vi "Label Generation.vi"(8 "error in":errorcluster, 10 "Resistance Value":string[](array[string]), 11 "Serial No":string) -> (0 "error out":errorcluster, 1 "Print Data":T1, 2 "Printer Command":string, 3 "QR data":string, 4 "error out 2":errorcluster)   [LabVIEW 2021]
uses:
  Gen fgv action.ctl
panel:
  out "Printer Command Out":string
  out "bytes written":i32
  in  "error in (no error)":errorcluster
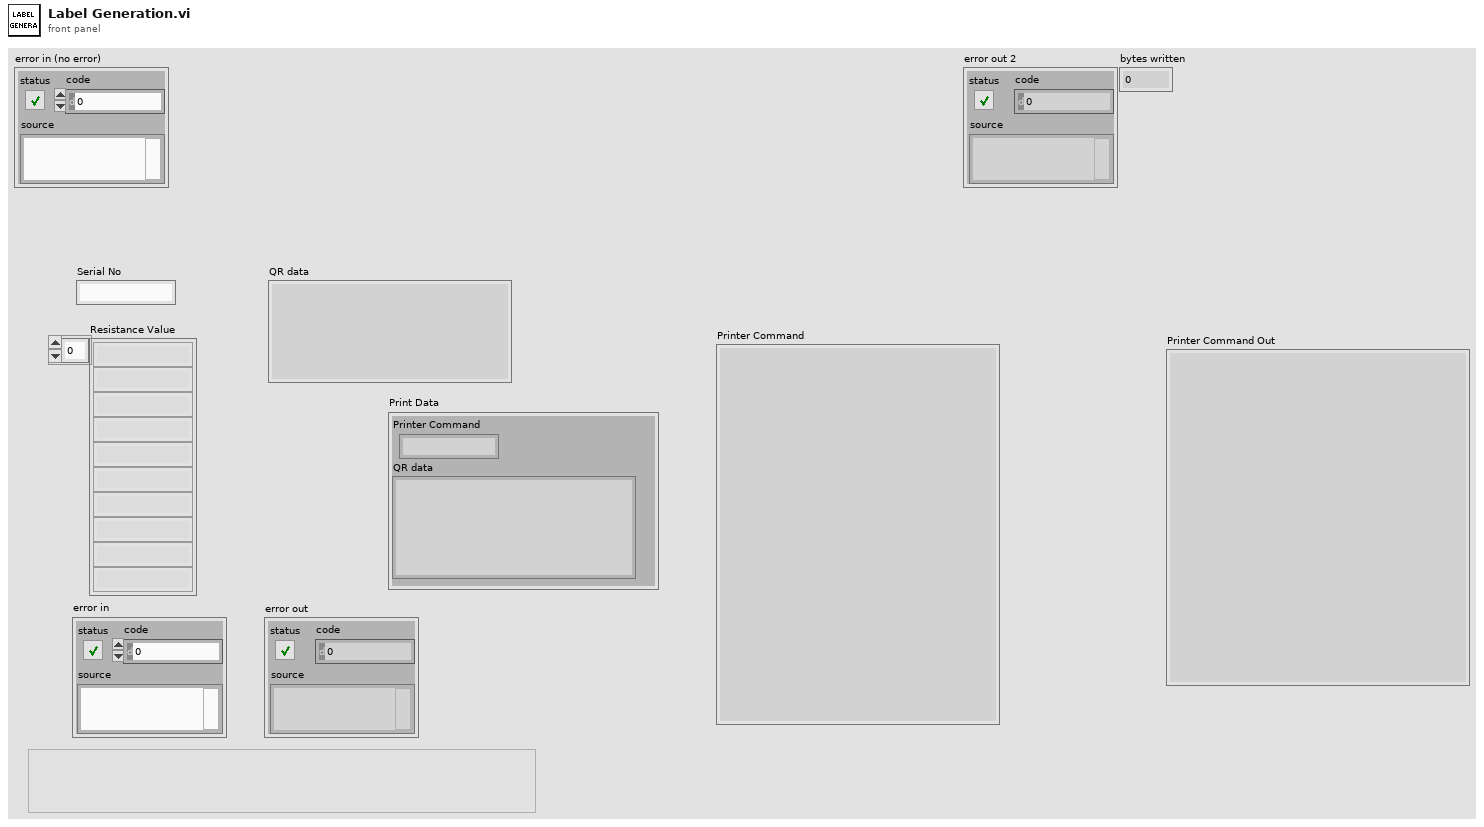
[diagram p1: front panel]
types:
  T1 = cluster{"Printer Command":string, "QR data":string}
  T2 = typedef "Gen FGV Action.ctl" = enum16{"Initialize", "Get Data", "Update Data", "Clear Data"}
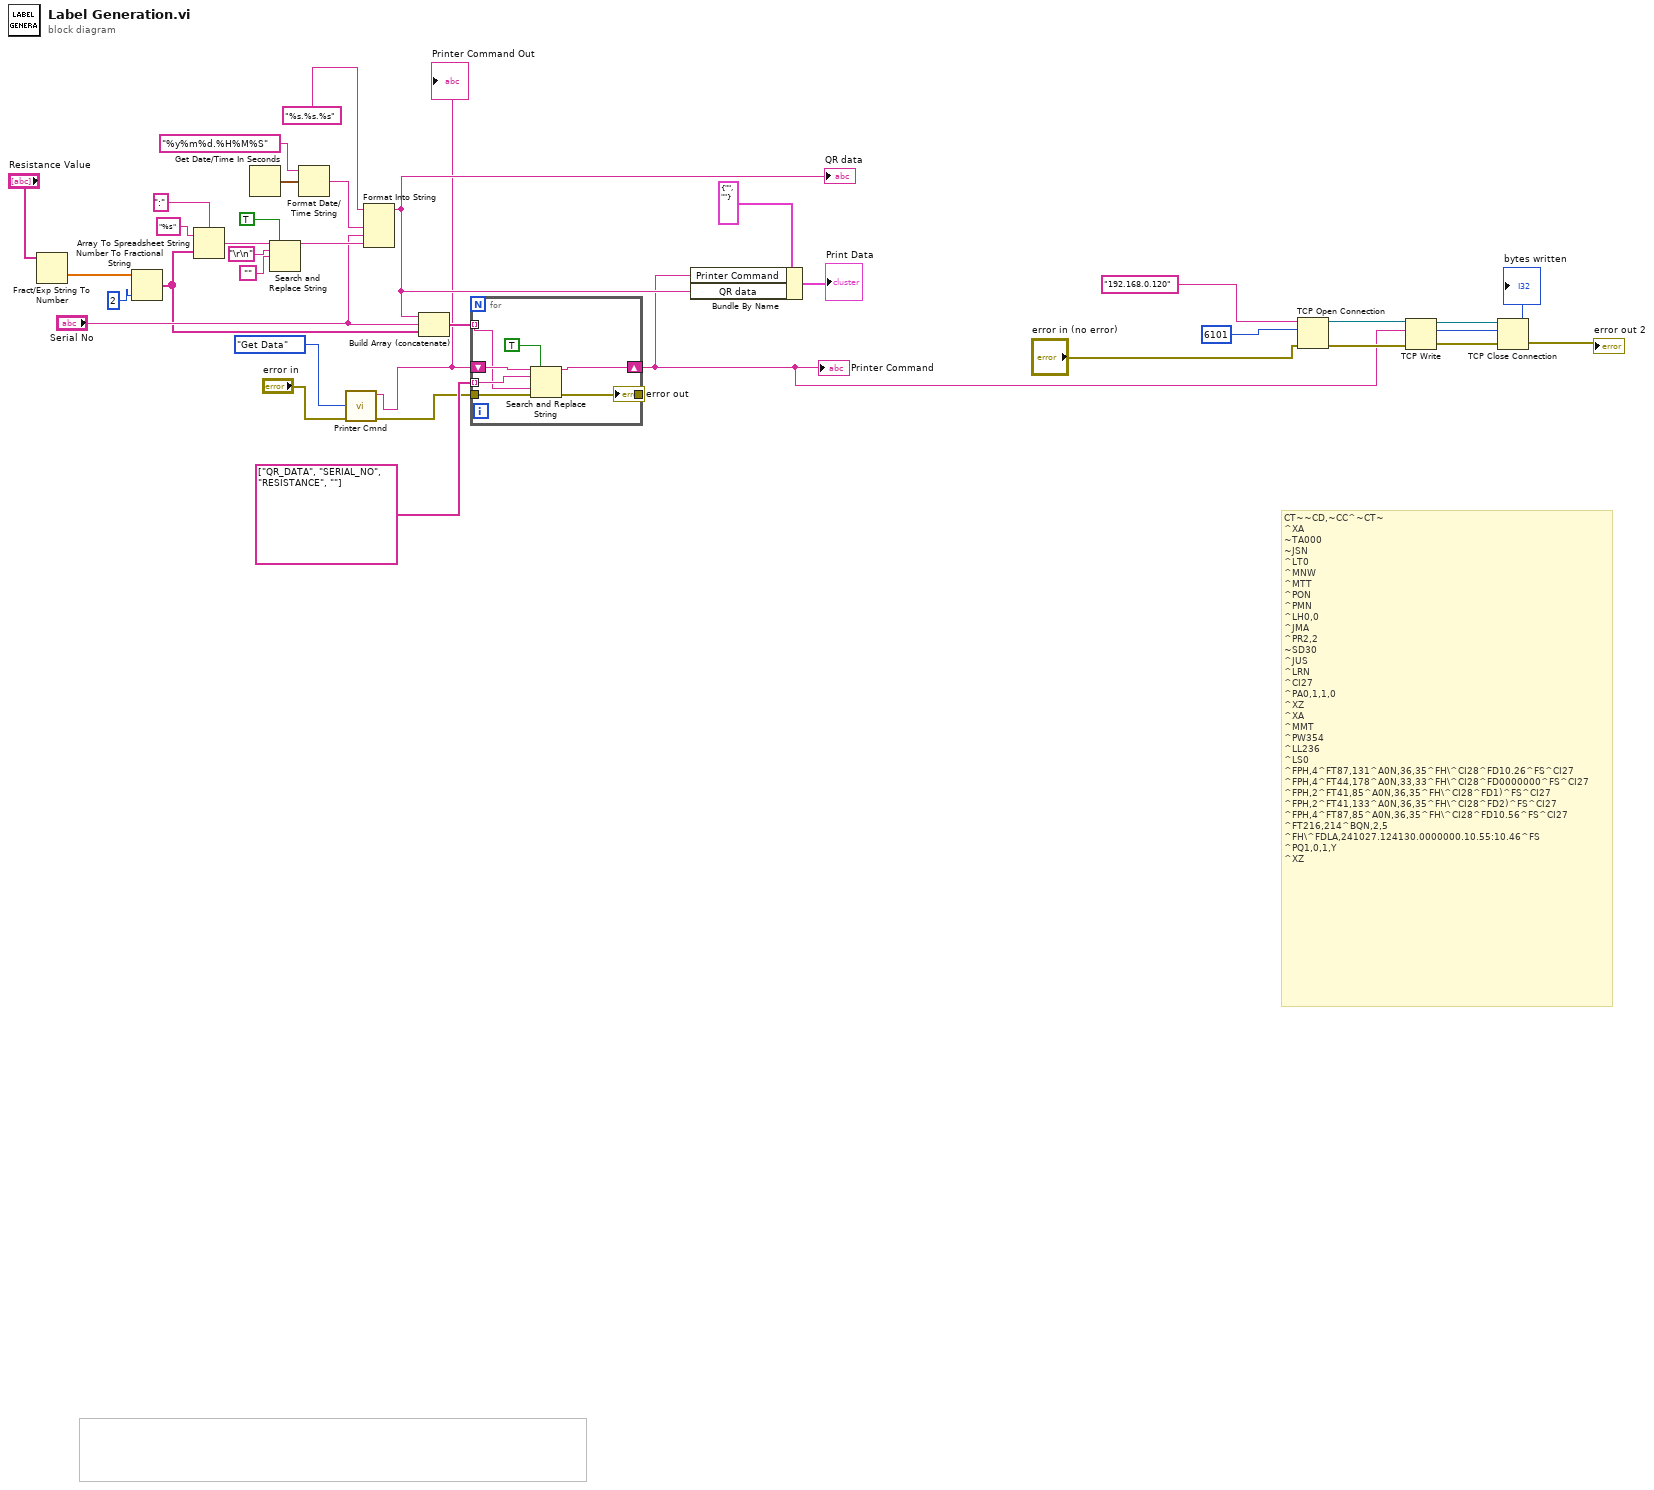
[diagram p0: block diagram]
diagram:
  # "CT~~CD,~CC^~CT~\n^XA\n~TA000\n~JSN\n^LT0\n^MNW\n^MTT\n^PON\n^PMN\n^LH0,0\n^JMA\n^PR2,2\n~SD30\n^JUS\n^LRN\n^CI27\n^PA0,1,1,0\n^XZ\n^XA\n^MMT\n^PW354\n^LL236\n^LS0\n^FPH,4^FT87,131^A0N,36,35^FH\\^CI28^FD10.26^FS^CI27\n^FPH,4^FT44,178^A0N,33,33^FH\\^CI28^FD0000000^FS^CI27\n^FPH,2^FT41,85^A0N,36,35^FH\\^CI28^FD1)^FS^CI27\n^FPH,2^FT41,133^A0N,36,35^FH\\^CI28^FD2)^FS^CI27\n^FPH,4^FT87,85^A0N,36,35^FH\\^CI28^FD10.56^FS^CI27\n^FT216,214^BQN,2,5\n^FH\\^FDLA,241027.124130.0000000.10.55:10.46^FS\n^PQ1,0,1,Y\n^XZ"
  n1 = Fract/Exp String To Number(string="Resistance Value") -> (number=w5:dbl[])  [unwired: 3 in, 1 out]
  n2 = Number To Fractional String(number=w5, precision (6)=i16 2) -> (F-format string=w7:string[])  [unwired: 2 in]
  n3 = Array To Spreadsheet String(delimiter (Tab)=":", array=w7, 3:"%s" ("format string")) -> (spreadsheet string=w27:string)
  n4 = Get Date/Time In Seconds() -> (seconds since 1Jan1904=w35:timestamp)
  n5 = Search and Replace String(replace all?=TRUE ("replace all? (F)"), input string=w27, search string="\r\n", replace string="") -> (result string=w26:string)  [unwired: 4 in, 3 out]
  n6 = Format Date/Time String(time format string (%c)="%y%m%d.%H%M%S", seconds (now)=w35) -> (date/time string=w33:string)  [unwired: 1 in]
  n7 = call "Printer Cmnd.vi"("Action?"=Gen_FGV_Action."Get Data", "error in (no error)"="error in") -> ("error out"=w1:errorcluster, "Printer Command Out"=w4:string)  [unwired: 8 in]
  "Printer Command Out" <- w4
  n8 = Format Into String(format string="%s.%s.%s", w33, "Serial No", w26) -> (resulting string=w21:string)  [unwired: 2 in, 1 out]
  "QR data" <- w21
  n9 = Build Array (concatenate)(w21, "Serial No", w7) -> (w30:string[])
  n10 = for {
    tunnel: w30 -> [w38] mode=indexing
    tunnel: w1 -> [w42]
    shift-right: [w40] -> w9
    shift-left: w4 -> [w41]
    tunnel: string[] ["QR_DATA", "SERIAL_NO", "RESISTANCE", ""] ("Array 2") -> [w39] mode=indexing
    tunnel: [w37] -> w28
    n11 = Search and Replace String(replace all?=TRUE ("replace all? (F)"), input string=w41, search string=w39, replace string=w38, error in=w42) -> (result string=w40:string, error out=w37:errorcluster)  [unwired: 3 in, 2 out]
  }
  "Printer Command" <- w9
  "error out" <- w28
  n12 = Bundle By Name(cluster=T1 {"Printer Command"="", "QR data"=""} ("Print Data"), "Printer Command"=w9, "QR data"=w21) -> (→"Print Data":T1)
  n13 = TCP Open Connection(address="192.168.0.120", remote port or service name=u16 6101, error in (no error)="error in (no error)") -> (connection ID=w17:refnum<k5>, error out=w13:errorcluster)  [unwired: 2 in]
  n14 = TCP Write(connection ID=w17, data in=w9, error in (no error)=w13) -> (connection ID out=w16:refnum<k5>, bytes written=→"bytes written":i32, error out=w12:errorcluster)  [unwired: 1 in]
  n15 = TCP Close Connection(connection ID=w16, error in (no error)=w12) -> (error out=→"error out 2":errorcluster)  [unwired: 1 in, 1 out]
